vi "PlotPressureAtGraph.vi"(9 "Press In":dbl, 10 "Array":dbl[][](array[numeric]), 11 "reference":refnum<vi>) -> (2 "Array Out":dbl[][](array[numeric]))   [LabVIEW 2013, in "main.lvlib"]
uses:
  main.lvlib
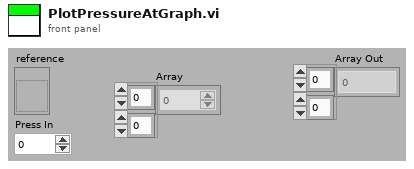
[diagram p1: front panel]
types:
  T1 = cluster{"Font Name:":string, "Size":i16, "Strikeout?":bool, "Italic?":bool, "Underline?":bool, "Outline?":bool, "Shadow?":bool, "Bold?":bool}
  T2 = enum16{"User-specified Font", "Application Font", "System Font", "Dialog Font"}
  T3 = cluster{"horizontal":enum16{"left", "center", "right"}, "vertical":enum16{"top", "center", "bottom"}}
  T4 = typedef "LVRectTypeDef.ctl" = cluster{"Left":i16, "Top":i16, "Right":i16, "Bottom":i16}
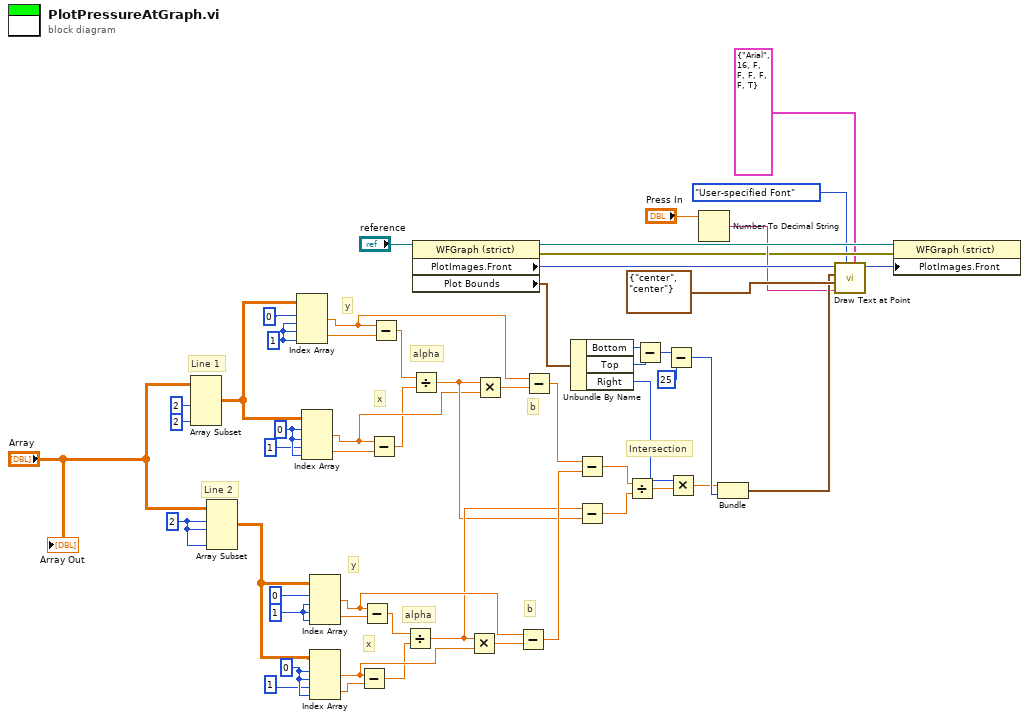
[diagram p0: block diagram]
diagram:
  w33 = 0
  w32 = 0
  w27 = 1 ("index (row)")
  w25 = 1 ("index (row)")
  w24 = 2
  # "Intersection"
  # "b"
  # "alpha"
  # "b"
  # "alpha"
  # "Line 2"
  # "Line 1"
  # "y"
  # "x"
  # "x"
  # "y"
  n1 = Array Subset(array="Array", length (row)=2 ("length"), length (col)=2 ("length")) -> (w34:dbl[][])  [unwired: 2 in]
  n2 = Array Subset(array="Array", index (row)=w24, length (row)=w24, length (col)=w24) -> (w35:dbl[][])  [unwired: 1 in]
  n3 = Index Array(array=w34, index (row) #1=0 ("disabled index (col)"), index (col) #1=w25, index (row) #2=w25, index (col) #2=w25) -> (element #1=w39:dbl, element #2=w40:dbl)
  n4 = Index Array(array=w34, index (row) #1=w33, index (col) #1=w33, index (row) #2=1 ("index"), index (col) #2=w33) -> (element #1=w42:dbl, element #2=w41:dbl)
  n5 = Index Array(array=w35, index (row) #1=0 ("index (row)"), index (col) #1=w27, index (row) #2=w27, index (col) #2=w27) -> (element #1=w53:dbl, element #2=w23:dbl)
  n6 = Index Array(array=w35, index (row) #1=w32, index (col) #1=w32, index (row) #2=1 ("index"), index (col) #2=w32) -> (element #1=w46:dbl, element #2=w29:dbl)
  n7 = Subtract(x=w46, y=w29) -> (x-y=w44:dbl)
  n8 = Subtract(x=w53, y=w23) -> (x-y=w45:dbl)
  n9 = Subtract(x=w42, y=w41) -> (x-y=w37:dbl)
  n10 = Subtract(x=w39, y=w40) -> (x-y=w36:dbl)
  n11 = Divide(x=w45, y=w44) -> (x/y=w50:dbl)
  n12 = Divide(x=w36, y=w37) -> (x/y=w49:dbl)
  n13 = property class="WFGraph (strict)"(reference="reference") -> (reference out=w17:refnum<vi>, error out=w11:errorcluster, "PlotImages.Front"=w18:picture, "Plot Bounds"=w15:T4)  [unwired: 1 in]
  n14 = Multiply(x=w50, y=w46) -> (x*y=w43:dbl)
  n15 = Multiply(x=w49, y=w42) -> (x*y=w38:dbl)
  n16 = Subtract(x=w53, y=w43) -> (x-y=w52:dbl)
  n17 = Subtract(x=w39, y=w38) -> (x-y=w51:dbl)
  n18 = Unbundle By Name(w15) -> ("Bottom"=w8:i16, "Top"=w7:i16, "Right"=w2:i16)
  n19 = Subtract(x=w51, y=w52) -> (x-y=w47:dbl)
  n20 = Subtract(x=w50, y=w49) -> (x-y=w48:dbl)
  n21 = Divide(x=w47, y=w48) -> (x/y=w3:dbl)
  n22 = Subtract(x=w8, y=w7) -> (x-y=w6:i16)
  n23 = Subtract(x=w6, y=i16 25) -> (x-y=w4:i16)
  n24 = Multiply(x=w2, y=w3) -> (x*y=w1:dbl)
  n25 = Number To Decimal String(number="Press In") -> (decimal integer string=w12:string)  [unwired: 1 in]
  n26 = Bundle(w1, w4) -> (w14:cluster{dbl, i16})  [unwired: 1 in]
  n27 = call <vilib>:"Draw Text at Point.vi"("[user-specified font]"=T1 {"Font Name:"="Arial", "Size"=16, "Strikeout?"=FALSE, "Italic?"=FALSE, "Underline?"=FALSE, "Outline?"=FALSE, "Shadow?"=FALSE, "Bold?"=TRUE}, "desired font(Application)"=T2."User-specified Font", "text"=w12, "alignment(left, top)"=T3 {"horizontal"=enum."center", "vertical"=enum."center"}, "origin"=w14, "picture"=w18) -> ("new picture"=w54:picture)  [unwired: 4 in, 1 out]
  n28 = property class="WFGraph (strict)"(reference=w17, error in=w11, "PlotImages.Front"=w54) -> ()  [unwired: 2 out]
  "Array Out" <- "Array"
